vi "Test Get VI Reference.vi"(8 "error in (no error)":errorcluster) -> (0 "error out":errorcluster)   [LabVIEW 2020, in "TEST JKI State Machine API.lvlib"]
uses:
  TEST JKI State Machine API.lvlib
  source/JKI SM/JKI SM.lvclass
  <vilib>/addons/_JKI Toolkits/Caraya/classes/Test/Test.lvclass
  <vilib>/addons/_JKI Toolkits/Caraya/classes/Assert/Assert.lvclass
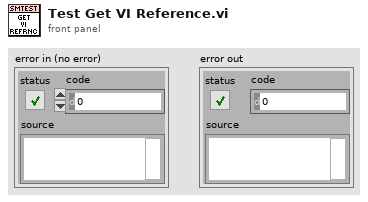
[diagram p1: front panel]
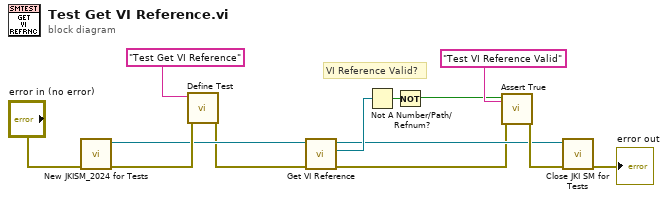
[diagram p0: block diagram]
diagram:
  # "VI Reference Valid?"
  n1 = call "New JKISM_2024 for Tests.vi"("error in (no error)"="error in (no error)") -> ("error out"=w8:errorcluster, "JKI SM out"=w4:refnum<class "JKI SM.lvclass">)  [unwired: 9 in]
  n2 = call <vilib>:"Define Test.vi"("error in (no error)"=w8, "Label (VI Title)"="Test Get VI Reference") -> ("error out"=w2:errorcluster)  [unwired: 8 in, 1 out]
  n3 = call "Get VI Reference.vi"("error in (no error)"=w2, "JKI SM in"=w4) -> ("error out"=w1:errorcluster, "VI"=w7:refnum<vi>, "JKI SM out"=w3:refnum<class "JKI SM.lvclass">)  [unwired: 7 in]
  n4 = Not A Number/Path/Refnum?(number/path/refnum=w7) -> (NaN/Path/Refnum?=w6:bool)
  n5 = Not(x=w6) -> (.not. x?=w5:bool)
  n6 = call <vilib>:"Assert True.vi"("Label"="Test VI Reference Valid", "error in (no error)"=w1, "True?"=w5) -> ("error out"=w11:errorcluster)  [unwired: 7 in, 1 out]
  n7 = call "Close JKI SM for Tests.vi"("error in (no error)"=w11, "JKI SM in"=w3) -> ("error out"=→"error out":errorcluster)  [unwired: 9 in]
